vi "Set DMM Function.vi"(8 "error in (no error)":errorcluster, 10 "Function":enum16{"AC Volts", "AC Current"}(ring), 11 "instrument handle":refnum<k15>) -> (0 "error out":errorcluster, 3 "instrument handle out":refnum<k15>)   [LabVIEW 2017]
uses:
  <instrlib>/niDMM/nidmm.llb/niDMM Function.ctl
  <instrlib>/niDMM/nidmm.llb/niDMM Resolution in Digits.ctl
  <instrlib>/niDMM/nidmm.llb/niDMM Configure Measurement Digits.vi
panel:
  in  "DMM Func":T1=enum."AC Current" caption="Function"
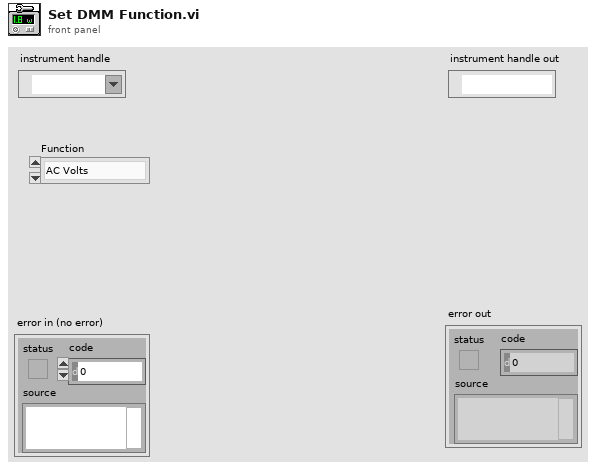
[diagram p1: front panel]
types:
  T1 = typedef "niDMM Function.ctl" = enum16{"DC Volts", "AC Volts", "DC Current", "AC Current", "2-wire Resistance", "4-wire Resistance", "Diode", "Frequency", "Period", "AC Volts DC Coupled", "Capacitance", "Inductance", "Temperature"}
  T2 = typedef "niDMM Resolution in Digits.ctl" = dbl
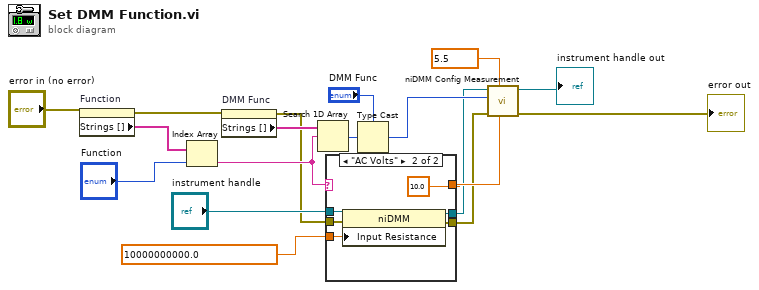
[diagram p0: block diagram]
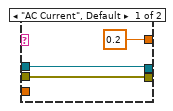
[diagram p2: hidden frame]
diagram:
  w2 = 10000000000.0 items=["1 M Ohm"=1000000.0, "10 M Ohm"=10000000.0, "Greater Than 10 G Ohm"=10000000000.0] ("Configuration:Measurement Options:Input Resistance")
  w9 = T2 5.5 items=["3 1/2"=3.5, "4 1/2"=4.5, "5 1/2"=5.5, "6 1/2"=6.5, "7 1/2"=7.5] ("Resolution in Digits")
  n1 = property on="Function" class="Enum (strict)"(error in="error in (no error)") -> (error out=w13:errorcluster, "Strings []"=w16:string[])  [unwired: 1 in, 1 out]
  n2 = Index Array(array=w16, index="Function") -> (element=w7:string)
  n3 = property on="DMM Func" class="Enum (strict)"(error in=w13) -> (error out=w3:errorcluster, "Strings []"=w12:string[])  [unwired: 1 in, 1 out]
  n4 = Search 1D Array(1D array=w12, element=w7) -> (index of element=w11:i32)  [unwired: 1 in]
  n5 = case shown="\"AC Volts\"" w7 {
    tunnel: [0.2 10.0] -> w6
    tunnel: "instrument handle" -> [w20 w26]
    tunnel: [w20 w25] -> w4
    tunnel: w3 -> [w19 w24]
    tunnel: w2 -> [_ w23]
    tunnel: [w19 w22] -> w1
    frame "AC Current", Default {
    }
    frame "AC Volts" {
      n6 = property class="niDMM"(reference=w26, error in=w24, "Input Resistance"=w23) -> (reference out=w25:refnum<k15>, error out=w22:errorcluster)
    }
  }
  n7 = Type Cast(type="DMM Func", x=w11) -> (*(type *) &x=w8:T1)
  n8 = call-poly <instrlib>:"niDMM Config Measurement.vi"("Range"=w6, "Resolution in Digits"=w9, "error in (no error)"=w1, "Function"=w8, "instrument handle"=w4) -> ("error out"=→"error out":errorcluster, "instrument handle out"=→"instrument handle out":refnum<k15>)  [unwired: 5 in]
